vi "Poll.vi"(0 "Fehler (Eingang, kein Fehler)":errorcluster, 5 "instanceHandle":u32, 7 "DLL-Path":path, 9 "maxValues":i32) -> (4 "Fehler (Ausgang)":errorcluster, 6 "instanceHandle":u32, 8 "DLL-Path":path, 10 "ERR_CODE":i32, 14 "scaledData":dbl[](array[numeric]), 15 "rawData":i32[](array[numeric]))   [LabVIEW 2015, in "MEDAQLib.lvlib"]
doc: "ERR_CODE Poll (DWORD instanceHandle, int *rawData, double *scaledData, int maxValues);\n\nGet the latest values from sensor."
uses:
  MEDAQLib.lvlib
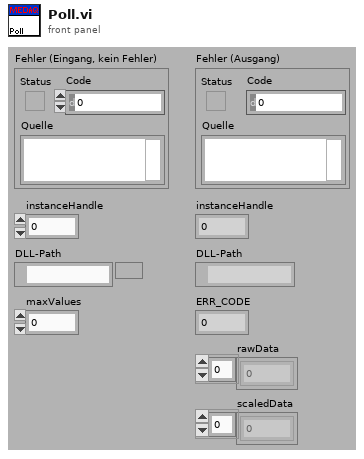
[diagram p1: front panel]
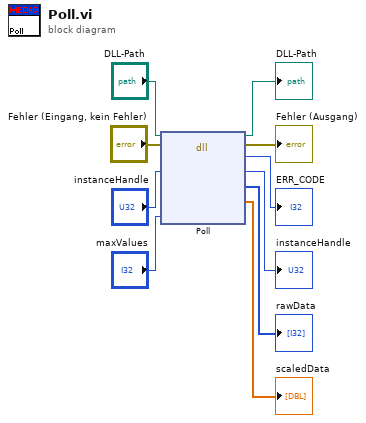
[diagram p0: block diagram]
diagram:
  n1 = dll-call lib="C:/Programme/National Instruments 8.6/LabVIEW 8.6/instr.lib/MEDAQLib/Release/MEDAQLib.dll" fn="Poll"(path in="DLL-Path", error in="Fehler (Eingang, kein Fehler)", "instanceHandle"="instanceHandle", "maxValues"="maxValues") -> (path out=→"DLL-Path":path, error out=→"Fehler (Ausgang)":errorcluster, "Rückgabetyp"=→"ERR_CODE":i32, "instanceHandle"=→"instanceHandle":u32, "rawData"=→"rawData":i32[], "scaledData"=→"scaledData":dbl[])  [unwired: 2 in, 2 out]
